vi "INIT_6517.vi"(9 "error in (no error)":errorcluster, 10 "VISA resource name":refnum<visa-resource-name>, 11 "Vin":dbl) -> (2 "error out":errorcluster, 3 "Vout":dbl)   [LabVIEW 2017]
uses:
  <instrlib>/Keithley 6517/Keithley 6517.lvlib
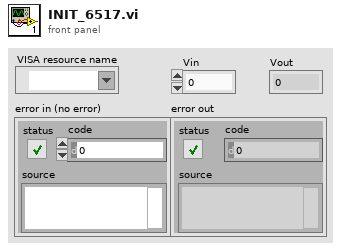
[diagram p1: front panel]
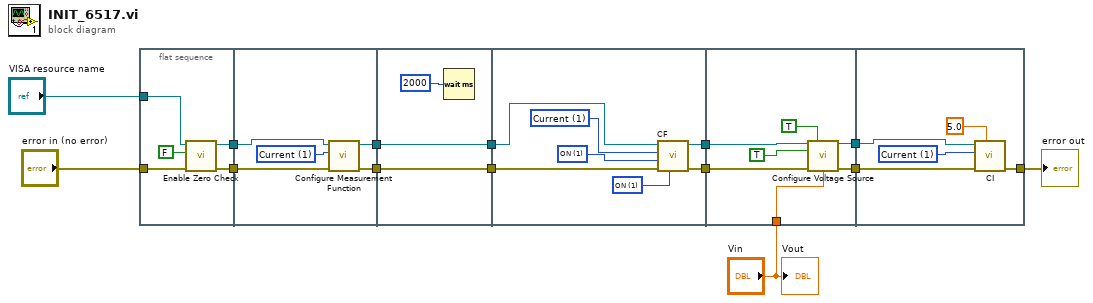
[diagram p0: block diagram]
diagram:
  n1 = flat-sequence {
    tunnel: "error in (no error)" -> [w16]
    tunnel: "VISA resource name" -> [w18]
    tunnel: [w19] -> w14
    tunnel: [w15] -> w13
    tunnel: w14 -> [w23]
    tunnel: [w24] -> w12
    tunnel: w13 -> [w21]
    tunnel: [w20] -> w11
    tunnel: w12 -> [w26]
    tunnel: [w26] -> w10
    tunnel: w11 -> [w25]
    tunnel: [w25] -> w9
    tunnel: w10 -> [w31]
    tunnel: [w30] -> w8
    tunnel: w9 -> [w29]
    tunnel: [w28] -> w7
    tunnel: w8 -> [w41]
    tunnel: [w40] -> w6
    tunnel: w7 -> [w39]
    tunnel: [w36] -> w5
    tunnel: "Vin" -> [w35]
    tunnel: w6 -> [w45]
    tunnel: w5 -> [w43]
    tunnel: [w42] -> w2
    frame #0 {
      n2 = call <instrlib>:"Enable Zero Check.vi"("error in (no error)"=w16, "Enable Zero Check (T: Enable)"=FALSE, "VISA resource name"=w18) -> ("error out"=w15:errorcluster, "VISA resource name out"=w19:refnum<visa-resource-name>)  [unwired: 7 in]
    }
    frame #1 {
      w22 = 1 items=["Voltage", "Current", "Resistance", "Charge"] ("Measurement Function (0: Voltage)")
      n3 = call <instrlib>:"Configure Measurement Function.vi"("error in (no error)"=w21, "Measurement Function (0: Voltage)"=w22, "VISA resource name"=w23) -> ("error out"=w20:errorcluster, "VISA resource name out"=w24:refnum<visa-resource-name>)  [unwired: 7 in]
    }
    frame #2 {
      n4 = Wait (ms)(milliseconds to wait=u32 2000 ("等待时间（毫秒）")) -> ()  [unwired: 1 out]
    }
    frame #3 {
      w32 = 1 items=["OFF", "ON", "ONCE"] ("Auto Resolution (1: ON)")
      w33 = 1 items=["OFF", "ON", "ONCE"] ("Auto Range (1: ON)")
      w34 = 1 items=["Voltage", "Current", "Resistance", "Charge"] ("Measurement Function (0: Voltage)")
      n5 = call "CF.vi"("Auto Resolution (1: ON)"=w32, "error in (no error)"=w29, "Auto Range (1: ON)"=w33, "Measurement Function (0: Voltage)"=w34, "VISA resource name"=w31) -> ("error out"=w28:errorcluster, "VISA resource name out"=w30:refnum<visa-resource-name>)  [unwired: 5 in]
    }
    frame #4 {
      n6 = call <instrlib>:"Configure Voltage Source.vi"("VISA resource name"=w41, "Enable LO Connection (F: Disable)"=TRUE, "Enable V-source (F: Disable)"=TRUE ("Operate ON"), "error in (no error)"=w39, "V-source Amplitude (0.000000E+0)"=w35) -> ("VISA resource name out"=w40:refnum<visa-resource-name>, "error out"=w36:errorcluster)  [unwired: 9 in]
    }
    frame #5 {
      w44 = 1 items=["Voltage", "Current", "Resistance", "Charge"] ("Measurement Function (0: Voltage)")
      n7 = call "CI.vi"("Integration Time (1 PLCs)"=5.0, "error in (no error)"=w43, "Measurement Function (0: Voltage)"=w44, "VISA resource name"=w45) -> ("error out"=w42:errorcluster)  [unwired: 6 in, 1 out]
    }
  }
  "error out" <- w2
  "Vout" <- "Vin"
